vi "Read xError_mm.vi"(8 "error in (no error)":errorcluster, 11 "GuiderMeasuredError in":refnum<class "GuiderMeasuredError.lvclass">) -> (0 "error out":errorcluster, 2 "xError_mm":dbl[unit] min=-1.0 max=1.0, 3 "GuiderMeasuredError out":refnum<class "GuiderMeasuredError.lvclass">)   [LabVIEW 2022 SP3, in "TCSDataDefinitions.lvlib" / "TCSGuiderCommand.lvlib" / "GuiderMeasuredError.lvclass"]
uses:
  GuiderMeasuredError.lvclass
  GuiderMeasuredError.lvclass/GuiderMeasuredError.ctl
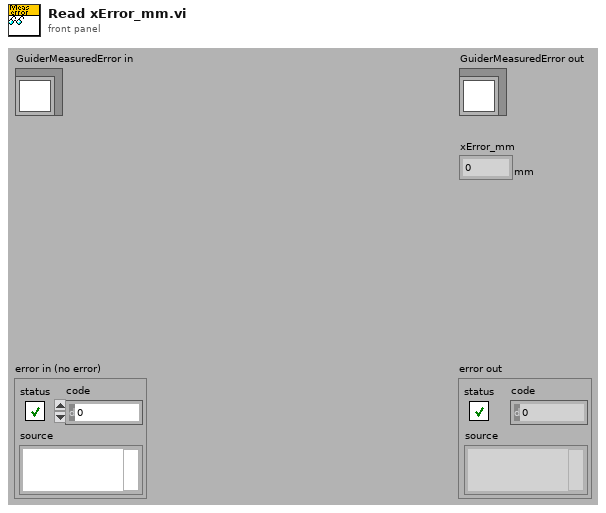
[diagram p1: front panel]
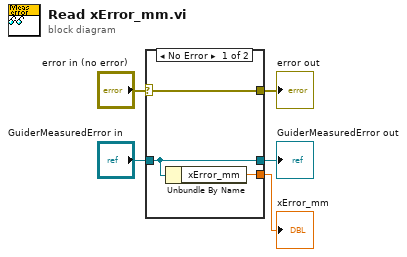
[diagram p0: block diagram]
diagram:
  n1 = case shown="No Error" "error in (no error)" {
    selector: "error in (no error)" -> [w8 w9]
    tunnel: [w8 w9] -> w4
    tunnel: [w7 w10] -> w2
    tunnel: "GuiderMeasuredError in" -> [w7 w10]
    tunnel: [w6 _] -> w1
    frame No Error {
      n2 = Unbundle By Name(w7) -> ("xError_mm"=w6:dbl[unit])
    }
    frame Error {
    }
  }
  "error out" <- w4
  "GuiderMeasuredError out" <- w2
  "xError_mm" <- w1
